vi "Is Done.vi"(8 "error in (no error)":errorcluster, 11 "Waveform in":refnum<class "Waveform.lvclass">) -> (0 "error out":errorcluster, 2 "Is Done":bool=TRUE, 3 "Waveform out":refnum<class "Waveform.lvclass">)   [LabVIEW 2015, in "Waveform.lvclass"]
uses:
  Waveform.lvclass
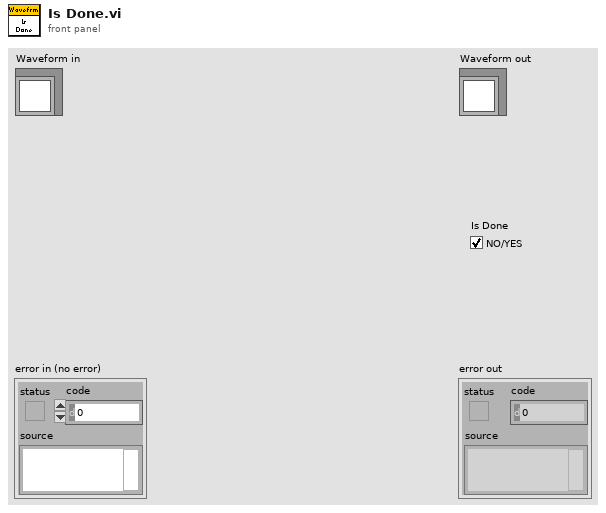
[diagram p1: front panel]
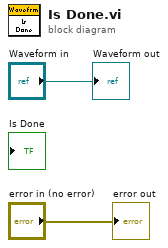
[diagram p0: block diagram]
diagram:
  "error out" <- "error in (no error)"
  "Waveform out" <- "Waveform in"
